vi "_attribute_read_int32.vi"(5 "Repeated Capability":string, 7 "Attribute":T1={"Identifier"="", "Descriptive Name"="", "Data Type"=enum."Integer 32", "Command"="", "Access"=enum."Read/Write", "Range Table"="", "Read Callback"="", "Write Callback"="", "Supported Models"="", "Instrument Options"="", "Index"=0, "OPC Wait"=FALSE, "No Status Check"=FALSE, "Cache Only"=FALSE}, 8 "error in":errorcluster caption="error in (no error)", 10 "Query Parameter":string, 11 "VISA resource name":refnum<visa-resource-name>) -> (0 "error out":errorcluster, 2 "Int32 out":i32, 3 "VISA resource name out":refnum<visa-resource-name>)   [LabVIEW 2020, in "Rohde&Schwarz RTx Oscilloscopes.lvlib" / "rsidr_core.lvlib"]
uses:
  rsidr_core.lvlib
  type_Attribute.ctl
  type_Attribute_Data_Type.ctl
  type_ReadWriteAccess.ctl
  Rohde&Schwarz RTx Oscilloscopes.lvlib
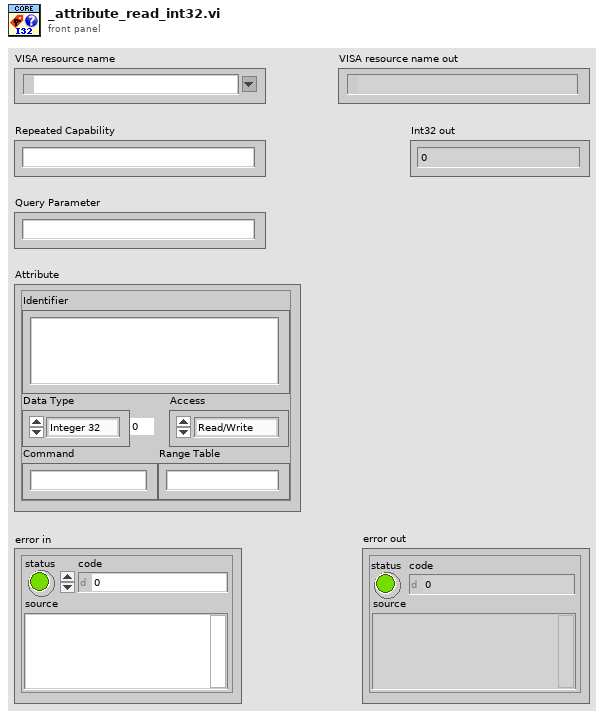
[diagram p1: front panel]
types:
  T1 = typedef "Rohde&Schwarz RTx Oscilloscopes.lvlib/rsidr_core.lvlib/type_Attribute.ctl" = cluster{"Identifier":string, "Descriptive Name":string, "Data Type":T2, "Command":string, "Access":T3, "Range Table":string, "Read Callback":string, "Write Callback":string, "Supported Models":string, "Instrument Options":string, "Index":i32, "OPC Wait":bool, "No Status Check":bool, "Cache Only":bool}
  T2 = typedef "Rohde&Schwarz RTx Oscilloscopes.lvlib/rsidr_core.lvlib/type_Attribute_Data_Type.ctl" = enum16{"Integer 32", "Double", "String", "Boolean", "None", "Integer 64", "RawString"}
  T3 = typedef "Rohde&Schwarz RTx Oscilloscopes.lvlib/rsidr_core.lvlib/type_ReadWriteAccess.ctl" = enum16{"Read Only", "Write Only", "Read/Write"}
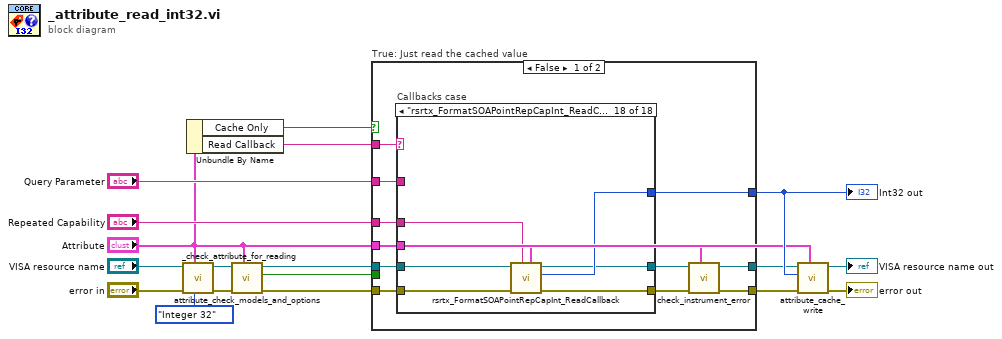
[diagram p0: block diagram]
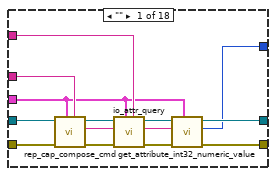
[diagram p2: hidden frame]
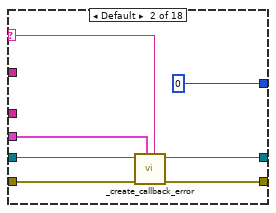
[diagram p3: hidden frame]
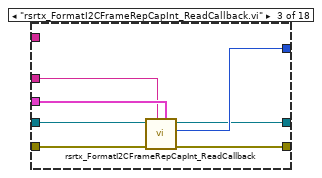
[diagram p4: hidden frame]
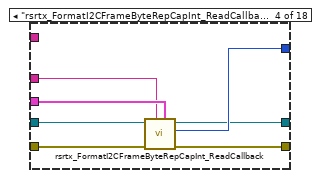
[diagram p5: hidden frame]
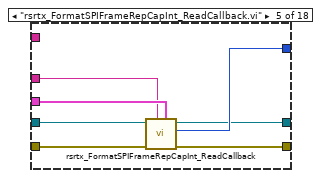
[diagram p6: hidden frame]
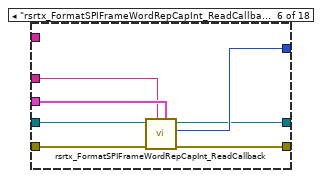
[diagram p7: hidden frame]
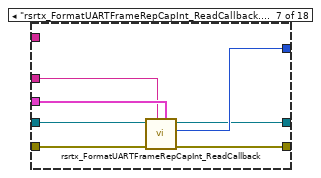
[diagram p8: hidden frame]
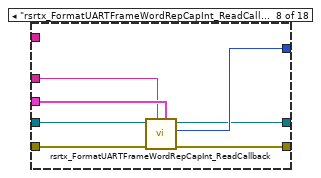
[diagram p9: hidden frame]
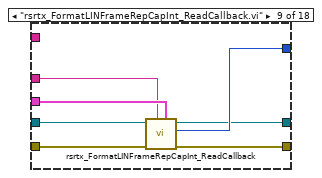
[diagram p10: hidden frame]
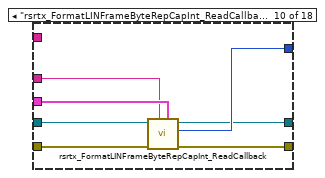
[diagram p11: hidden frame]
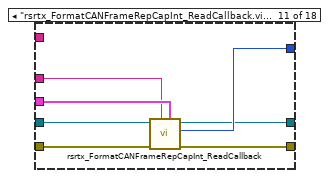
[diagram p12: hidden frame]
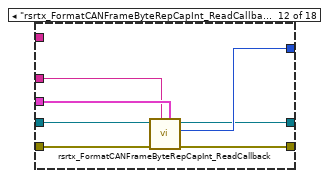
[diagram p13: hidden frame]
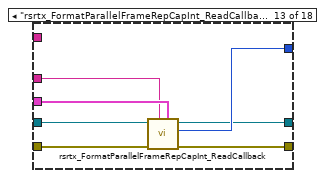
[diagram p14: hidden frame]
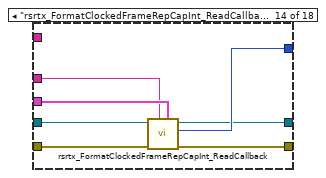
[diagram p15: hidden frame]
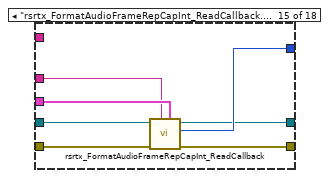
[diagram p16: hidden frame]
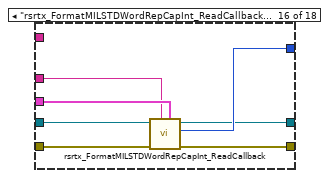
[diagram p17: hidden frame]
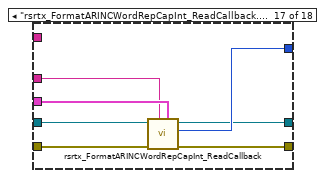
[diagram p18: hidden frame]
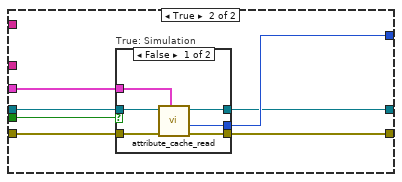
[diagram p19: hidden frame]
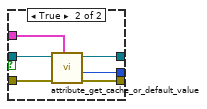
[diagram p20: hidden frame]
diagram:
  n1 = call "_check_attribute_for_reading.vi"("Expected Data Type"=type_Attribute_Data_Type."Integer 32" ("Data Type"), "Attribute"="Attribute", "error in"="error in", "VISA resource name"="VISA resource name") -> ("error out"=w9:errorcluster, "VISA resource name out"=w8:refnum<visa-resource-name>)  [unwired: 6 in]
  n2 = Unbundle By Name("Attribute") -> ("Cache Only"=w1:bool, "Read Callback"=w10:string)
  n3 = call "attribute_check_models_and_options.vi"("Attribute"="Attribute", "error in"=w9, "VISA resource name"=w8) -> ("error out"=w7:errorcluster, "Simulation Mode"=w5:bool, "VISA resource name out"=w6:refnum<visa-resource-name>)  [unwired: 6 in]
  n4 = case "True: Just read the cached value" shown="False" w1 {
    tunnel: "Repeated Capability" -> [w29 _]
    tunnel: [w21 w165] -> w4
    tunnel: [w20 w164] -> w3
    tunnel: [w28 w166] -> w13
    tunnel: w10 -> [w27 _]
    tunnel: w6 -> [w26 w168]
    tunnel: w7 -> [w25 w169]
    tunnel: "Attribute" -> [w19 w167]
    tunnel: "Query Parameter" -> [w24 _]
    tunnel: w5 -> [_ w163]
    frame False {
      n5 = case "Callbacks case" shown="\"rsrtx_FormatSOAPointRepCapInt_ReadCallback.vi\"" w27 {
        selector: w27 -> [_ w45 _ _ _ _ _ _ _ _ _ _ _ _ _ _ _ _]
        tunnel: w26 -> [w43 w49 w56 w63 w70 w77 w84 w91 w98 w105 w112 w119 w126 w133 w140 w147 w154 w161]
        tunnel: w25 -> [w42 w50 w57 w64 w71 w78 w85 w92 w99 w106 w113 w120 w127 w134 w141 w148 w155 w162]
        tunnel: w29 -> [w36 _ w54 w61 w68 w75 w82 w89 w96 w103 w110 w117 w124 w131 w138 w145 w152 w159]
        tunnel: [w41 w47 w51 w58 w65 w72 w79 w86 w93 w100 w107 w114 w121 w128 w135 w142 w149 w156] -> w22
        tunnel: [w40 w48 w52 w59 w66 w73 w80 w87 w94 w101 w108 w115 w122 w129 w136 w143 w150 w157] -> w23
        tunnel: [w33 0 ("Attribute Value I32") w53 w60 w67 w74 w81 w88 w95 w102 w109 w116 w123 w130 w137 w144 w151 w158] -> w28
        tunnel: w19 -> [w30 w46 w55 w62 w69 w76 w83 w90 w97 w104 w111 w118 w125 w132 w139 w146 w153 w160]
        tunnel: w24 -> [w31 _ _ _ _ _ _ _ _ _ _ _ _ _ _ _ _ _]
        frame "" {
          n6 = call "rep_cap_compose_cmd.vi"("Repeated Capability"=w36, "Attribute"=w30, "error in"=w42, "VISA resource name"=w43) -> ("error out"=w39:errorcluster, "Command out"=w38:string, "VISA resource name out"=w37:refnum<visa-resource-name>)  [unwired: 5 in]
          n7 = call "io_attr_query.vi"("Query Parameter (None)"=w31, "Attribute"=w30, "error in"=w39, "write buffer"=w38, "VISA resource name"=w37) -> ("error out"=w35:errorcluster, "read buffer"=w32:string, "VISA resource name out"=w34:refnum<visa-resource-name>)  [unwired: 4 in]
          n8 = call "get_attribute_int32_numeric_value.vi"("Attribute"=w30, "error in"=w35, "Cmd Value in"=w32, "VISA resource name"=w34) -> ("error out"=w40:errorcluster, "Int32 value out"=w33:i32, "VISA resource name out"=w41:refnum<visa-resource-name>)  [unwired: 5 in]
        }
        frame Default {
          n9 = call "_create_callback_error.vi"("Callback Name"=w45, "Attribute"=w46, "error in"=w50, "VISA resource name"=w49) -> ("error out"=w48:errorcluster, "VISA resource name out"=w47:refnum<visa-resource-name>)  [unwired: 6 in]
        }
        frame "rsrtx_FormatI2CFrameRepCapInt_ReadCallback.vi" {
          n10 = call "rsrtx_FormatI2CFrameRepCapInt_ReadCallback.vi"("Attribute"=w55, "Repeated Capability"=w54, "error in"=w57, "VISA resource name"=w56) -> ("error out"=w52:errorcluster, "Attribute Value I32"=w53:i32, "VISA resource name out"=w51:refnum<visa-resource-name>)  [unwired: 5 in]
        }
        frame "rsrtx_FormatI2CFrameByteRepCapInt_ReadCallback.vi" {
          n11 = call "rsrtx_FormatI2CFrameByteRepCapInt_ReadCallback.vi"("Attribute"=w62, "Repeated Capability"=w61, "error in"=w64, "VISA resource name"=w63) -> ("error out"=w59:errorcluster, "Attribute Value I32"=w60:i32, "VISA resource name out"=w58:refnum<visa-resource-name>)  [unwired: 5 in]
        }
        frame "rsrtx_FormatSPIFrameRepCapInt_ReadCallback.vi" {
          n12 = call "rsrtx_FormatSPIFrameRepCapInt_ReadCallback.vi"("Attribute"=w69, "Repeated Capability"=w68, "error in"=w71, "VISA resource name"=w70) -> ("error out"=w66:errorcluster, "Attribute Value I32"=w67:i32, "VISA resource name out"=w65:refnum<visa-resource-name>)  [unwired: 5 in]
        }
        frame "rsrtx_FormatSPIFrameWordRepCapInt_ReadCallback.vi" {
          n13 = call "rsrtx_FormatSPIFrameWordRepCapInt_ReadCallback.vi"("Attribute"=w76, "Repeated Capability"=w75, "error in"=w78, "VISA resource name"=w77) -> ("error out"=w73:errorcluster, "Attribute Value I32"=w74:i32, "VISA resource name out"=w72:refnum<visa-resource-name>)  [unwired: 5 in]
        }
        frame "rsrtx_FormatUARTFrameRepCapInt_ReadCallback.vi" {
          n14 = call "rsrtx_FormatUARTFrameRepCapInt_ReadCallback.vi"("Attribute"=w83, "Repeated Capability"=w82, "error in"=w85, "VISA resource name"=w84) -> ("error out"=w80:errorcluster, "Attribute Value I32"=w81:i32, "VISA resource name out"=w79:refnum<visa-resource-name>)  [unwired: 5 in]
        }
        frame "rsrtx_FormatUARTFrameWordRepCapInt_ReadCallback.vi" {
          n15 = call "rsrtx_FormatUARTFrameWordRepCapInt_ReadCallback.vi"("Attribute"=w90, "Repeated Capability"=w89, "error in"=w92, "VISA resource name"=w91) -> ("error out"=w87:errorcluster, "Attribute Value I32"=w88:i32, "VISA resource name out"=w86:refnum<visa-resource-name>)  [unwired: 5 in]
        }
        frame "rsrtx_FormatLINFrameRepCapInt_ReadCallback.vi" {
          n16 = call "rsrtx_FormatLINFrameRepCapInt_ReadCallback.vi"("Attribute"=w97, "Repeated Capability"=w96, "error in"=w99, "VISA resource name"=w98) -> ("error out"=w94:errorcluster, "Attribute Value I32"=w95:i32, "VISA resource name out"=w93:refnum<visa-resource-name>)  [unwired: 5 in]
        }
        frame "rsrtx_FormatLINFrameByteRepCapInt_ReadCallback.vi" {
          n17 = call "rsrtx_FormatLINFrameByteRepCapInt_ReadCallback.vi"("Attribute"=w104, "Repeated Capability"=w103, "error in"=w106, "VISA resource name"=w105) -> ("error out"=w101:errorcluster, "Attribute Value I32"=w102:i32, "VISA resource name out"=w100:refnum<visa-resource-name>)  [unwired: 5 in]
        }
        frame "rsrtx_FormatCANFrameRepCapInt_ReadCallback.vi" {
          n18 = call "rsrtx_FormatCANFrameRepCapInt_ReadCallback.vi"("Attribute"=w111, "Repeated Capability"=w110, "error in"=w113, "VISA resource name"=w112) -> ("error out"=w108:errorcluster, "Attribute Value I32"=w109:i32, "VISA resource name out"=w107:refnum<visa-resource-name>)  [unwired: 5 in]
        }
        frame "rsrtx_FormatCANFrameByteRepCapInt_ReadCallback.vi" {
          n19 = call "rsrtx_FormatCANFrameByteRepCapInt_ReadCallback.vi"("Attribute"=w118, "Repeated Capability"=w117, "error in"=w120, "VISA resource name"=w119) -> ("error out"=w115:errorcluster, "Attribute Value I32"=w116:i32, "VISA resource name out"=w114:refnum<visa-resource-name>)  [unwired: 5 in]
        }
        frame "rsrtx_FormatParallelFrameRepCapInt_ReadCallback.vi" {
          n20 = call "rsrtx_FormatParallelFrameRepCapInt_ReadCallback.vi"("Attribute"=w125, "Repeated Capability"=w124, "error in"=w127, "VISA resource name"=w126) -> ("error out"=w122:errorcluster, "Attribute Value I32"=w123:i32, "VISA resource name out"=w121:refnum<visa-resource-name>)  [unwired: 5 in]
        }
        frame "rsrtx_FormatClockedFrameRepCapInt_ReadCallback.vi" {
          n21 = call "rsrtx_FormatClockedFrameRepCapInt_ReadCallback.vi"("Attribute"=w132, "Repeated Capability"=w131, "error in"=w134, "VISA resource name"=w133) -> ("error out"=w129:errorcluster, "Attribute Value I32"=w130:i32, "VISA resource name out"=w128:refnum<visa-resource-name>)  [unwired: 5 in]
        }
        frame "rsrtx_FormatAudioFrameRepCapInt_ReadCallback.vi" {
          n22 = call "rsrtx_FormatAudioFrameRepCapInt_ReadCallback.vi"("Attribute"=w139, "Repeated Capability"=w138, "error in"=w141, "VISA resource name"=w140) -> ("error out"=w136:errorcluster, "Attribute Value I32"=w137:i32, "VISA resource name out"=w135:refnum<visa-resource-name>)  [unwired: 5 in]
        }
        frame "rsrtx_FormatMILSTDWordRepCapInt_ReadCallback.vi" {
          n23 = call "rsrtx_FormatMILSTDWordRepCapInt_ReadCallback.vi"("Attribute"=w146, "Repeated Capability"=w145, "error in"=w148, "VISA resource name"=w147) -> ("error out"=w143:errorcluster, "Attribute Value I32"=w144:i32, "VISA resource name out"=w142:refnum<visa-resource-name>)  [unwired: 5 in]
        }
        frame "rsrtx_FormatARINCWordRepCapInt_ReadCallback.vi" {
          n24 = call "rsrtx_FormatARINCWordRepCapInt_ReadCallback.vi"("Attribute"=w153, "Repeated Capability"=w152, "error in"=w155, "VISA resource name"=w154) -> ("error out"=w150:errorcluster, "Attribute Value I32"=w151:i32, "VISA resource name out"=w149:refnum<visa-resource-name>)  [unwired: 5 in]
        }
        frame "rsrtx_FormatSOAPointRepCapInt_ReadCallback.vi" {
          n25 = call "rsrtx_FormatSOAPointRepCapInt_ReadCallback.vi"("Attribute"=w160, "Repeated Capability"=w159, "error in"=w162, "VISA resource name"=w161) -> ("error out"=w157:errorcluster, "Attribute Value I32"=w158:i32, "VISA resource name out"=w156:refnum<visa-resource-name>)  [unwired: 5 in]
        }
      }
      n26 = call "check_instrument_error.vi"("Attribute"=w19, "error in"=w23, "VISA resource name"=w22) -> ("error out"=w21:errorcluster, "VISA resource name out"=w20:refnum<visa-resource-name>)  [unwired: 7 in]
    }
    frame True {
      n27 = case "True: Simulation" shown="False" w163 {
        tunnel: w169 -> [w175 w181]
        tunnel: w168 -> [w174 w180]
        tunnel: w167 -> [w173 w176]
        tunnel: [w172 w177] -> w166
        tunnel: [w171 w179] -> w165
        tunnel: [w170 w178] -> w164
        frame False {
          n28 = call "attribute_cache_read.vi"("Attribute"=w173, "error in"=w175, "VISA resource name"=w174) -> ("error out"=w171:errorcluster, "Int32 out"=w172:i32, "VISA resource name out"=w170:refnum<visa-resource-name>)  [unwired: 1 in, 5 out]
        }
        frame True {
          n29 = call "attribute_get_cache_or_default_value.vi"("Attribute"=w176, "error in"=w181, "VISA resource name"=w180) -> ("error out"=w179:errorcluster, "Int32 out"=w177:i32, "VISA resource name out"=w178:refnum<visa-resource-name>)  [unwired: 1 in, 5 out]
        }
      }
    }
  }
  "Int32 out" <- w13
  n30 = call "attribute_cache_write.vi"("Attribute"="Attribute", "error in"=w4, "Value in"=w13, "VISA resource name"=w3) -> ("error out"=→"error out":errorcluster, "VISA resource name out"=→"VISA resource name out":refnum<visa-resource-name>)  [unwired: 6 in]
